vi "VariantToProperties.vi"(0 "NHRDCPower in":refnum<class "NHRDCPower.lvclass">, 11 "error in (no error)":errorcluster) -> (4 "NHRDCPower out":refnum<class "NHRDCPower.lvclass">, 6 "NHRDC":T3 {"Modules"."Regulation Gain (1=100%)" min=0.0 max=1.0; "Modules"."OutputSettings"."Wait on Value" items=["Voltage Greater Than Or Equal To", "Voltage Less Than Or Equal To", "Current Greater Than Or Equal To", "Current Less Than Or Equal To", "Power Greater Than Or Equal To", "Power Less Than Or Equal To"]; "Modules"."operating state (Off)" items=["Off", "Stand By", "Charge", "Discharge", "Battery Emulation"]}, 8 "Meas":T2, 10 "MeasName":string, 13 "Measurement Refresh Time (ms)":u32, 14 "Modules":T1 {"Regulation Gain (1=100%)" min=0.0 max=1.0; "OutputSettings"."Wait on Value" items=["Voltage Greater Than Or Equal To", "Voltage Less Than Or Equal To", "Current Greater Than Or Equal To", "Current Less Than Or Equal To", "Power Greater Than Or Equal To", "Power Less Than Or Equal To"]; "operating state (Off)" items=["Off", "Stand By", "Charge", "Discharge", "Battery Emulation"]}, 15 "error out":errorcluster)   [LabVIEW 2018, in "AcPwrPlugins.lvlib" / "NHRDCPower.lvclass"]
doc: "This VI exposes the Device Settings, Measurement Refresh Time, Measurement Settings, and Modules properties from the variant that they were stored in."
uses:
  NHRDCPower.lvclass
  C:/Projects/ICDAS - Local tetsing/NistPluggableModules/AcPwr/AcPwrPlugins/AcPwrBaseClass/AcPwrBase.lvclass
  TypeDefs/Device(s)Settings.ctl
  TypeDefs/Modules.ctl
  TypeDefs/Measurements.ctl
  AcPwrBaseClass/AcPwrBase.lvclass/AcPwrBase.ctl
  AcPwrBaseClass/Accessors/Read BaseConfig.vi
panel:
  out "VTP Time":u32
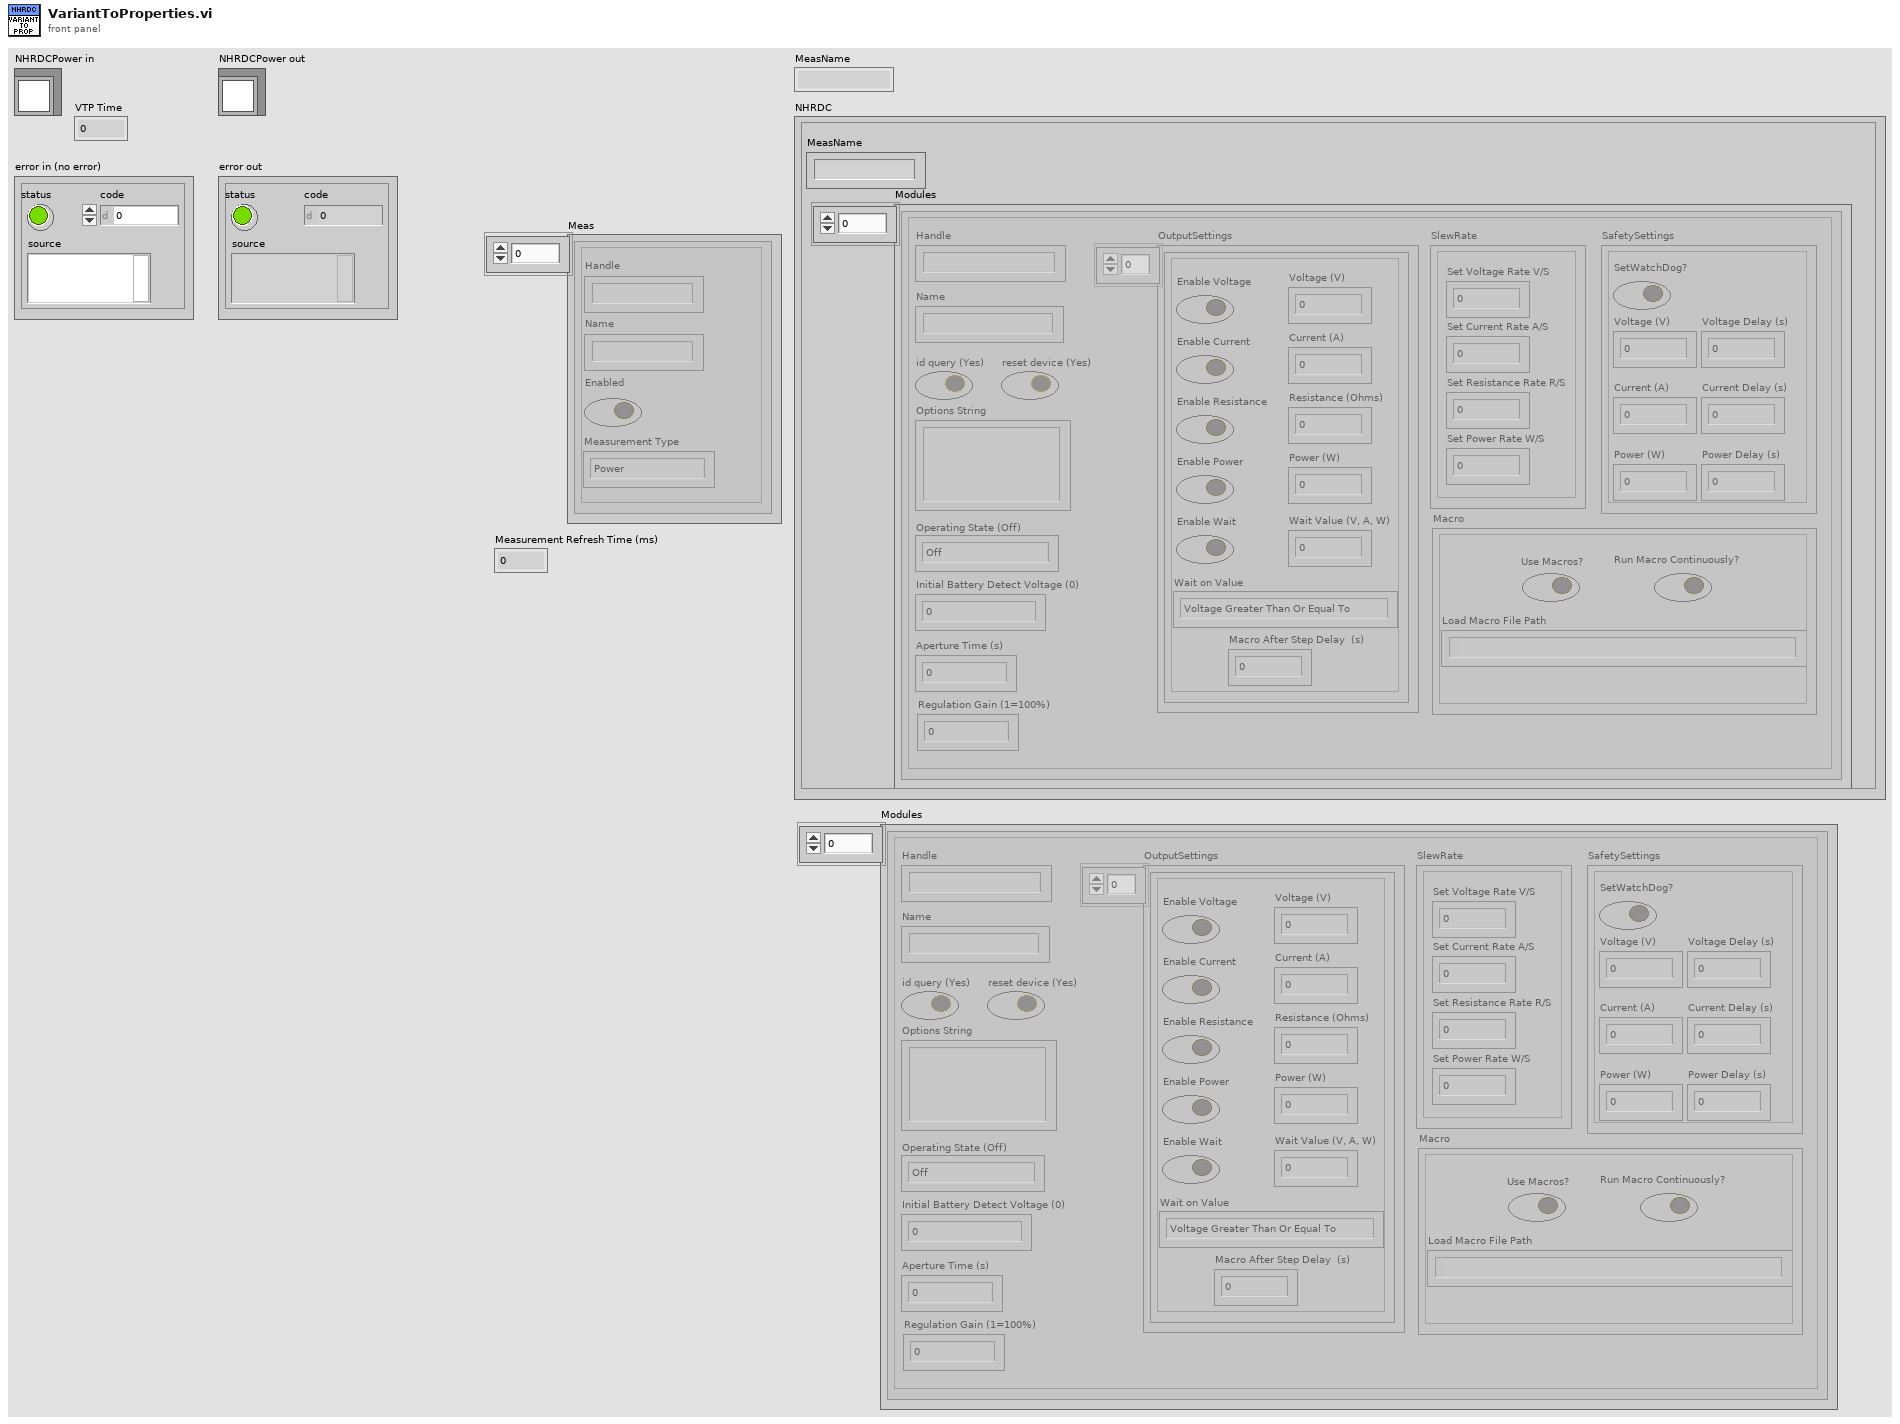
[diagram p1: front panel]
types:
  T1 = typedef "AcPwrPlugins.lvlib/NHRDCPower.lvclass/Modules.ctl" = cluster{"Handle":string, "Name":string, "id query (Yes)":bool, "reset device (Yes)":bool, "Connected":bool, "Initial Battery Detect Voltage (0)":dbl, "SafetySettings":cluster{"SetWatchDog?":bool, "Voltage (V)":dbl, "Current (A)":dbl, "Power (W)":dbl, "Voltage Delay (s)":dbl, "Current Delay (s)":dbl, "Power Delay (s)":dbl}, "Options String":string, "Aperture Time (s)":dbl, "operating state (Off)":i32, "OutputSettings":cluster{"Voltage (V)":dbl, "Current (A)":dbl, "Resistance (Ohms)":dbl, "Power (W)":dbl, "Enable Voltage":bool, "Enable Current":bool, "Enable Resistance":bool, "Enable Power":bool, "Macro After Step Delay  (s)":dbl, "Wait Value (V, A, W)":dbl, "Enable Wait":bool, "Wait on Value":i32}[], "SlewRate":cluster{"Set Voltage Rate V/S":dbl, "Set Current Rate A/S":dbl, "Set Resistance Rate R/S":dbl, "Set Power Rate W/S":dbl}, "Macro":cluster{"Save Macro?":bool, "Load Macro From File?":bool, "Run Macro Continuously?":bool, "Use Macros?":bool, "Load Macro File Path":path, "Save Macro File Path":string}, "Regulation Gain (1=100%)":dbl, "UpdatingOntheFly":bool}[]
  T2 = typedef "AcPwrPlugins.lvlib/NHRDCPower.lvclass/Measurements.ctl" = cluster{"Handle":string, "Name":string, "Enabled":bool, "Measurement Value":sgl, "Measurement Type":enum16{"Power", "Current", "Voltage"}}[]
  T3 = typedef "AcPwrPlugins.lvlib/NHRDCPower.lvclass/Device(s)Settings.ctl" = cluster{"MeasName":string, "Modules":T1}
  T4 = typedef "AcPwrPlugins.lvlib/AcPwrBase.lvclass/BaseConfig.ctl" = cluster{"Frequency":dbl, "FrequencyRange":dbl[], "Phases":T5[], "Name":string, "PluginConfigVariant":variant, "PluginMeasVariant":variant}
  T5 = typedef "AcPwrPlugins.lvlib/AcPwrBase.lvclass/Phase.ctl" = cluster{"Name":string, "Enabled":bool, "VoltageLevel":dbl, "Handle":string, "VoltageRange":dbl[], "Connected":bool, "CurrentLimit":dbl, "Waveform":string}
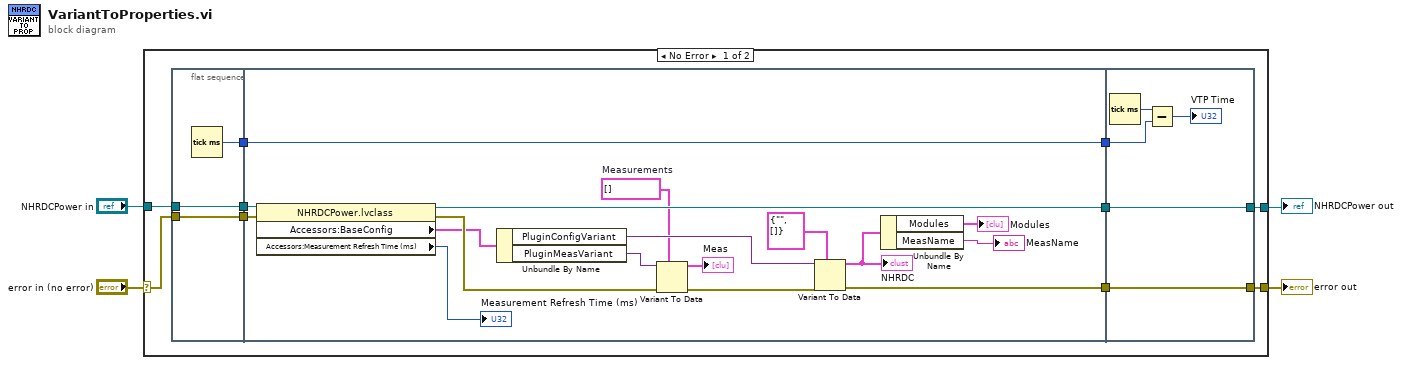
[diagram p0: block diagram]
diagram:
  n1 = case shown="No Error" "error in (no error)" {
    selector: "error in (no error)" -> [w12 w41]
    tunnel: [w14 w41] -> w2
    tunnel: "NHRDCPower in" -> [w13 w40]
    tunnel: [w11 w40] -> w3
    frame No Error {
      n2 = flat-sequence {
        tunnel: w12 -> [w16]
        tunnel: w13 -> [w17]
        tunnel: [w17] -> w8
        tunnel: [w16] -> w7
        tunnel: [w15] -> w5
        tunnel: [w34] -> w10
        tunnel: [w31] -> w9
        tunnel: w8 -> [w33]
        tunnel: w7 -> [w32]
        tunnel: [w18] -> w6
        tunnel: w5 -> [w18]
        tunnel: [w38] -> w11
        tunnel: [w39] -> w14
        tunnel: w10 -> [w39]
        tunnel: w9 -> [w38]
        tunnel: w6 -> [w36]
        frame #0 {
          n3 = Tick Count (ms)() -> (millisecond timer value=w15:u32)
        }
        frame #1 {
          w23 = T2 []  # Measurements
          n4 = property class="NHRDCPower.lvclass"(reference=w33, error in=w32) -> (reference out=w31:refnum<class "NHRDCPower.lvclass">, error out=w26:errorcluster, "Accessors:BaseConfig"=w20:T4, "Accessors:Measurement Refresh Time (ms)"=→"Measurement Refresh Time (ms)":u32)
          n5 = Unbundle By Name(w20) -> ("PluginConfigVariant"=w30:variant, "PluginMeasVariant"=w24:variant)
          n6 = Variant To Data(error in=w26, type=w23, Variant=w24) -> (data=→"Meas":T2, error out=w25:errorcluster)
          n7 = Variant To Data(error in=w25, type=T3 {"MeasName"="", "Modules"=[]} ("Device(s)Settings"), Variant=w30) -> (data=w28:T3, error out=w34:errorcluster)
          "NHRDC" <- w28
          n8 = Unbundle By Name(w28) -> ("Modules"=→"Modules":T1, "MeasName"=→"MeasName":string)
        }
        frame #2 {
          n9 = Tick Count (ms)() -> (millisecond timer value=w37:u32)
          n10 = Subtract(x=w37, y=w36) -> (x-y=→"VTP Time":u32)
        }
      }
    }
    frame Error {
    }
  }
  "error out" <- w2
  "NHRDCPower out" <- w3
